vi "Process.vi"(8 "error in":errorcluster, 11 "Plugin in":refnum<class "Test Sequencer.lvclass">) -> (0 "error out":errorcluster, 3 "Plugin out":refnum<class "Test Sequencer.lvclass">)   [LabVIEW 2023, in "Test Sequencer.lvlib" / "Test Sequencer.lvclass"]
uses:
  Test Sequencer.lvclass
  C:/Program Files/National Instruments/LabVIEW 2023/vi.lib/FlexLogger/SDK/PluginSDK.lvlibp/PEFClasses/SDK/Plugin/Plugin.lvclass
  Test Sequencer.lvclass/Test Sequencer.ctl
  <vilib>/FlexLogger/SDK/PluginSDK.lvlibp/PEFClasses/SDK/Plugin/DataHelpers/Write 2D DBL (NChan NSamples).vi
  <vilib>/FlexLogger/SDK/PluginSDK.lvlibp/PEFClasses/SDK/Plugin/Plugin.lvclass
  C:/Program Files/National Instruments/LabVIEW 2023/vi.lib/FlexLogger/SDK/PluginSDK.lvlibp/PEFClasses/SDK/Processing Element/Processing Element.lvclass
  C:/Users/bbuchana/Documents/LabVIEW Projects/FlexLogger IO Plug-ins/Test Sequencer/Test Sequencer.lvclass
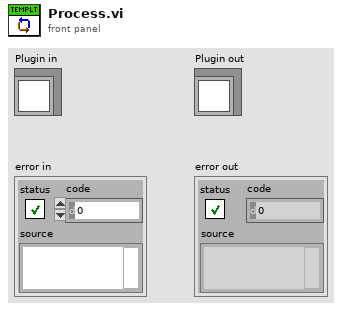
[diagram p1: front panel]
types:
  T1 = typedef "Params.ctl" = cluster{"Sequence Durations":dbl[], "Reset on Test Start":bool, "Current Sequence ID":u32, "Total Iterations":u32, "Last Timestamp":timestamp, "Number of Sequence Steps":i32}
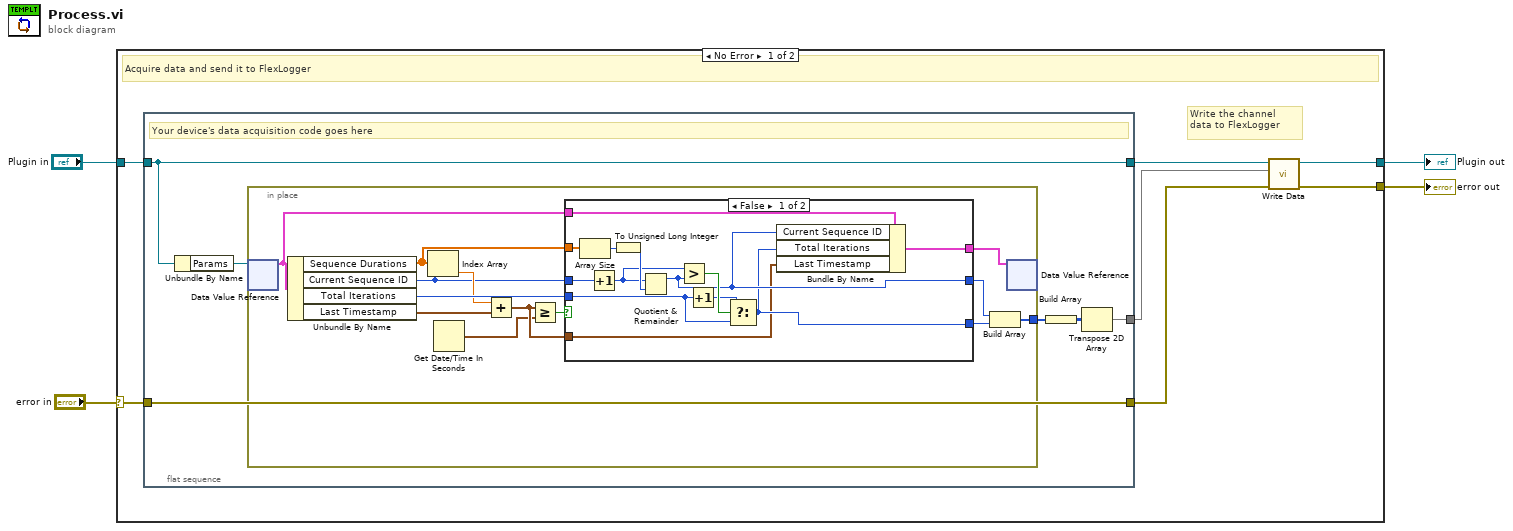
[diagram p0: block diagram]
diagram:
  n1 = case shown="No Error" "error in" {
    selector: "error in" -> [w10 w47]
    tunnel: [w6 w48] -> w4
    tunnel: "Plugin in" -> [w11 w48]
    tunnel: [w7 w47] -> w1
    frame No Error {
      # "Write the channel data to FlexLogger"
      # "Acquire data and send it to FlexLogger"
      n2 = flat-sequence {
        tunnel: [w12] -> w5
        tunnel: w11 -> [w16]
        tunnel: [w16] -> w9
        tunnel: w10 -> [w17]
        tunnel: [w17] -> w8
        frame #0 {
          # "Your device's data acquisition code goes here"
          n3 = Unbundle By Name(w16) -> ("Params"=w15:refnum<data-value>)
          n4 = in-place {
            in-place-border: [w27] -> w14
            n5 = in-place-dvr #1(w15) -> (w30:T1)  [unwired: 1 out]
            n6 = Unbundle By Name(w30) -> ("Sequence Durations"=w29:dbl[], "Current Sequence ID"=w23:u32, "Total Iterations"=w28:u32, "Last Timestamp"=w20:timestamp)
            n7 = Index Array(array=w29, index=w23) -> (element=w24:dbl)
            n8 = Get Date/Time In Seconds() -> (seconds since 1Jan1904=w22:timestamp)
            n9 = Add(x=w24, y=w20) -> (x+y=w25:timestamp)
            n10 = Greater Or Equal?(x=w25, y=w22) -> (x >= y?=w21:bool)
            n11 = case shown="False" w21 {
              tunnel: w30 -> [w37 w44]
              tunnel: w23 -> [w41 w46]
              tunnel: w29 -> [w43 _]
              tunnel: w28 -> [w39 w45]
              tunnel: [w35 w46] -> w19
              tunnel: [w34 w45] -> w18
              tunnel: [w36 w44] -> w26
              tunnel: w25 -> [w31 _]
              frame False {
                n12 = Array Size(array=w43) -> (size(s)=w42:i32)
                n13 = Increment(x=w41) -> (x+1=w32:u32)
                n14 = To Unsigned Long Integer(number=w42) -> (unsigned 32bit integer=w33:u32)
                n15 = Quotient & Remainder(x=w32, y=w33) -> (x-y*floor(x/y)=w35:u32)  [unwired: 1 out]
                n16 = Greater?(x=w32, y=w35) -> (0:w40:bool)
                n17 = Increment(x=w39) -> (x+1=w38:u32)
                n18 = Select(t=w38, s=w40, f=w39) -> (s? t:f=w34:u32)
                n19 = Bundle By Name(cluster=w37, "Current Sequence ID"=w35, "Total Iterations"=w34, "Last Timestamp"=w31) -> (w36:T1)
              }
              frame True {
              }
            }
            n20 = Build Array(w19, w18) -> (w27:u32[])
            n21 = in-place-dvr #1(w26) -> ()  [unwired: 2 out]
          }
          n22 = Build Array(w14) -> (w13:u32[][])
          n23 = Transpose 2D Array(2D array=w13) -> (transposed array=w12:u32[][])
        }
      }
      n24 = call-poly <vilib>:"Write Data.vi"("error in (no error)"=w8, "Data"=w5, "Plugin in"=w9) -> ("error out"=w7:errorcluster, "Plugin out"=w6:refnum<class "Test Sequencer.lvclass">)  [unwired: 7 in]
    }
    frame Error {
    }
  }
  "error out" <- w1
  "Plugin out" <- w4
